vi "SetLogFormatter.vi"(8 "Error in (no error)":errorcluster, 10 "LogFormatterInterface in":refnum<class "LogFormatterInterface.lvclass">, 11 "LogWriterStream in":refnum<class "LogWriterStream.lvclass">) -> (0 "Error out":errorcluster, 3 "LogWriterStream out":refnum<class "LogWriterStream.lvclass">)   [LabVIEW 2011, in "LogWriterStream.lvclass"]
uses:
  LogWriterStream.lvclass
  Formatter/LogFormatterInterface/LogFormatterInterface.lvclass
  LogWriterInterface/LogWriterInterface.lvclass
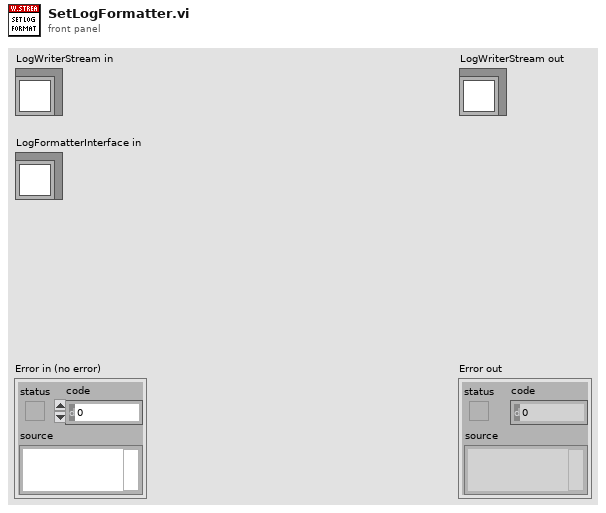
[diagram p1: front panel]
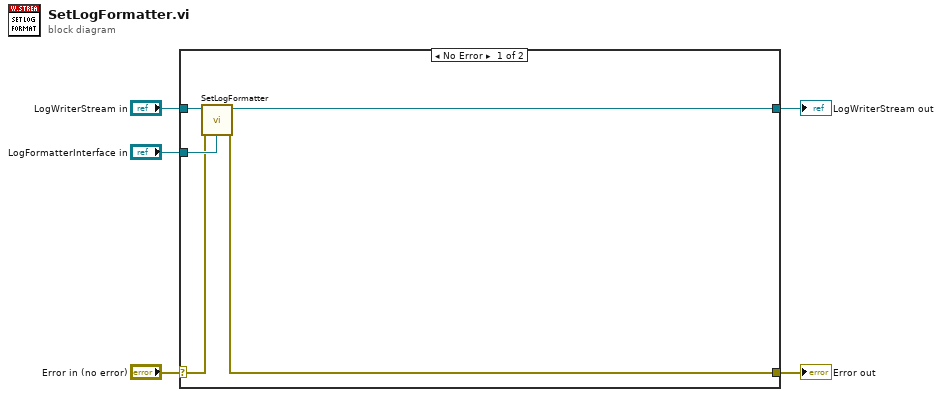
[diagram p0: block diagram]
diagram:
  n1 = case shown="No Error" "Error in (no error)" {
    selector: "Error in (no error)" -> [w7 w12]
    tunnel: [w6 w12] -> w4
    tunnel: [w9 w11] -> w2
    tunnel: "LogWriterStream in" -> [w10 w11]
    tunnel: "LogFormatterInterface in" -> [w8 _]
    frame No Error {
      n2 = call-parent "SetLogFormatter.vi"("Error in (no error)"=w7, "LogFormatterInterface in"=w8, "LogWriterInterface in"=w10) -> ("Error out"=w6:errorcluster, "LogWriterInterface out"=w9:refnum<class "LogWriterStream.lvclass">)  [unwired: 7 in]
    }
    frame Error {
    }
  }
  "Error out" <- w4
  "LogWriterStream out" <- w2
